vi "read buffer.vi"(8 "error in (no error)":errorcluster, 11 "Data Buffer in":refnum<class "Data Buffer.lvclass">) -> (0 "error out":errorcluster, 2 "XY Graph":T1(array[cluster]), 3 "Data Buffer out":refnum<class "Data Buffer.lvclass">)   [LabVIEW 2022 SP3, in "Data Buffer.lvclass"]
uses:
  Data Buffer.lvclass
  Data Buffer.lvclass/Data Buffer.ctl
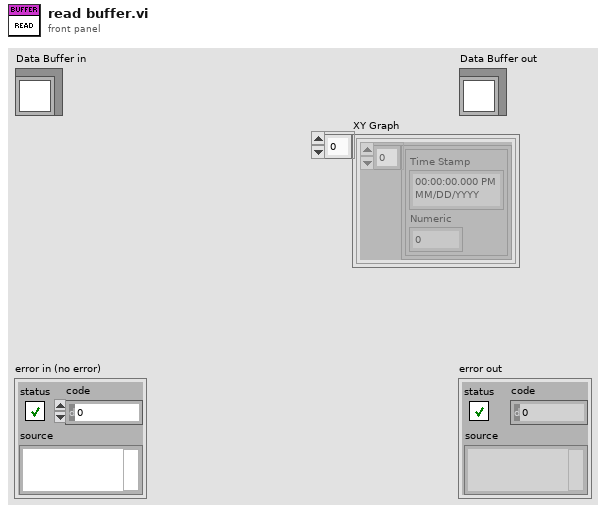
[diagram p1: front panel]
types:
  T1 = cluster{cluster{"Time Stamp":timestamp, "Numeric":dbl}[]}[]
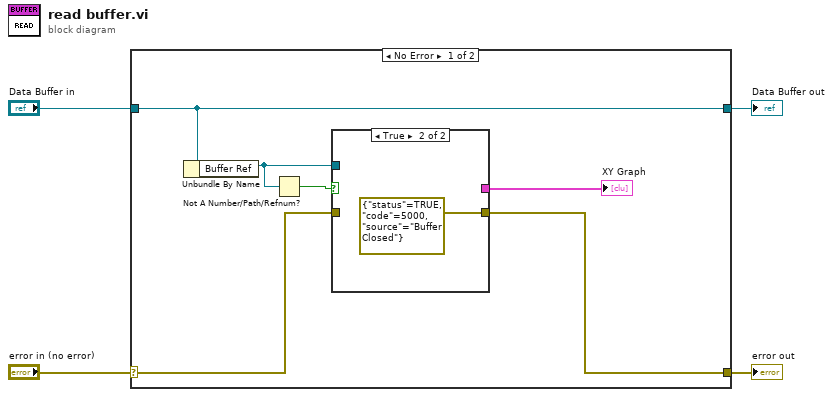
[diagram p0: block diagram]
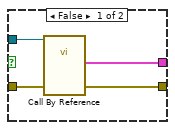
[diagram p2: hidden frame]
diagram:
  n1 = case shown="No Error" "error in (no error)" {
    selector: "error in (no error)" -> [w8 w17]
    tunnel: [w7 w17] -> w3
    tunnel: [w10 w16] -> w1
    tunnel: "Data Buffer in" -> [w10 w16]
    frame No Error {
      n2 = Unbundle By Name(w10) -> ("Buffer Ref"=w6:refnum<vi>)
      n3 = Not A Number/Path/Refnum?(number/path/refnum=w6) -> (NaN/Path/Refnum?=w5:bool)
      n4 = case shown="True" w5 {
        tunnel: [w14 _] -> w9
        tunnel: w8 -> [w13 _]
        tunnel: [w12 errorcluster {"status"=TRUE, "code"=5000, "source"="Buffer Closed"} ("error out")] -> w7
        tunnel: w6 -> [w11 _]
        frame False {
          n5 = call-by-ref "?"(reference=w11, "error in (no error)"=w13) -> ("error out"=w12:errorcluster, "XY Graph"=w14:T1)  [unwired: 10 in, 2 out]
        }
        frame True {
        }
      }
      "XY Graph" <- w9
    }
    frame Error {
    }
  }
  "error out" <- w3
  "Data Buffer out" <- w1
